vi "posi incial-proceso 5.vi"() -> ()   [LabVIEW 2020]
panel:
  out "posi incial-proceso 5":T1
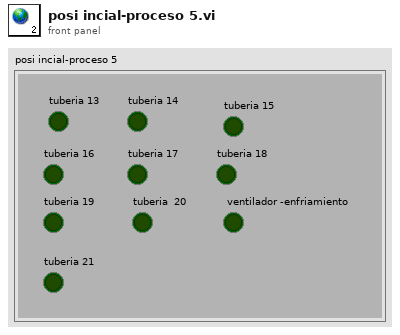
[diagram p1: front panel]
types:
  T1 = cluster{"tuberia 13":bool, "tuberia 14":bool, "tuberia 15":bool, "tuberia 16":bool, "tuberia 17":bool, "tuberia 18":bool, "tuberia 19":bool, "tuberia  20":bool, " ventilador -enfriamiento":bool, "tuberia 21":bool}
diagram:
